vi "Display History.vi"(11 "Discard Deck":variant[](array[variant])) -> (2 "Array Size Error?":bool)   [LabVIEW 2019]
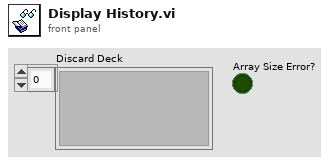
[diagram p1: front panel]
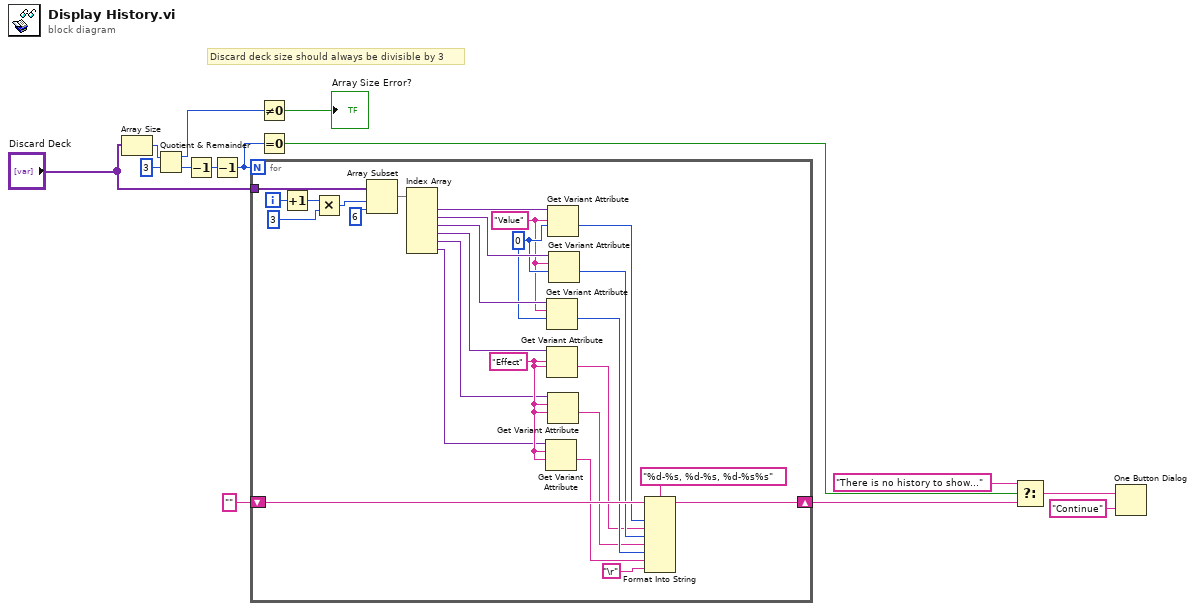
[diagram p0: block diagram]
diagram:
  # "Discard deck size should always be divisible by 3"
  n1 = Array Size(array="Discard Deck") -> (size(s)=w12:i32)
  n2 = Quotient & Remainder(x=w12, y=3) -> (x-y*floor(x/y)=w11:i32, floor(x/y)=w6:i32)
  n3 = Decrement(x=w6) -> (x-1=w7:i32)
  n4 = Decrement(x=w7) -> (x-1=w5:i32)
  n5 = for {
    N: w5 -> [_]
    tunnel: "Discard Deck" -> [w33]
    shift-right: [w17] -> w1
    shift-left: "" ("name") -> [w26]
    i -> [w15]
    w30 = "Effect" ("name")
    w37 = 0 ("Value 1")
    w36 = "Value" ("name")
    n6 = Increment(x=w15) -> (x+1=w16:i32)
    n7 = Multiply(x=w16, y=3) -> (x*y=w31:i32)
    n8 = Array Subset(array=w33, index=w31, length=6 ("y")) -> (w32:variant[])
    n9 = Index Array(array=w32) -> (element #1=w38:variant, element #2=w39:variant, element #3=w40:variant, element #4=w29:variant, element #5=w28:variant, element #6=w27:variant)  [unwired: 6 in]
    n10 = Get Variant Attribute(Variant=w27, name=w30, default value (empty Variant)=w30) -> (value=w18:string)  [unwired: 1 in, 3 out]
    n11 = Get Variant Attribute(Variant=w40, name=w36, default value (empty Variant)=w37) -> (value=w21:i32)  [unwired: 1 in, 3 out]
    n12 = Get Variant Attribute(Variant=w29, name=w30, default value (empty Variant)=w30) -> (value=w20:string)  [unwired: 1 in, 3 out]
    n13 = Get Variant Attribute(Variant=w38, name=w36, default value (empty Variant)=w37) -> (value=w23:i32)  [unwired: 1 in, 3 out]
    n14 = Get Variant Attribute(Variant=w28, name=w30, default value (empty Variant)=w30) -> (value=w19:string)  [unwired: 1 in, 3 out]
    n15 = Get Variant Attribute(Variant=w39, name=w36, default value (empty Variant)=w37) -> (value=w22:i32)  [unwired: 1 in, 3 out]
    n16 = Format Into String(format string="%d-%s, %d-%s, %d-%s%s", initial string=w26, w23, w20, w22, w19, w21, w18, "\r") -> (resulting string=w17:string)  [unwired: 1 in, 1 out]
  }
  n17 = Not Equal To 0?(x=w11) -> (x != 0?=→"Array Size Error?":bool)
  n18 = Equal To 0?(x=w5) -> (x = 0?=w4:bool)
  n19 = Select(t="There is no history to show..." ("button name (\"OK\")"), s=w4, f=w1) -> (s? t:f=w2:string)
  n20 = One Button Dialog(message=w2, button name ("OK")="Continue") -> ()  [unwired: 1 out]
